vi "Corner Position to Bounds.vi"(10 "bottom right":T1, 11 "top left":T1) -> (3 "bounds":T2)   [LabVIEW 2010, in "NI_SE_Front Panel Layout.lvlib"]
uses:
  NI_SE_Front Panel Layout.lvlib
  <vilib>/Utility/miscctls.llb/LVRectTypeDef.ctl
  <vilib>/Utility/miscctls.llb/LVPointTypeDef.ctl
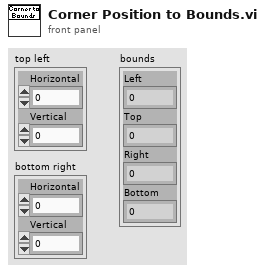
[diagram p1: front panel]
types:
  T1 = typedef "LVPointTypeDef.ctl" = cluster{"Horizontal":i16, "Vertical":i16}
  T2 = typedef "LVRectTypeDef.ctl" = cluster{"Left":i16, "Top":i16, "Right":i16, "Bottom":i16}
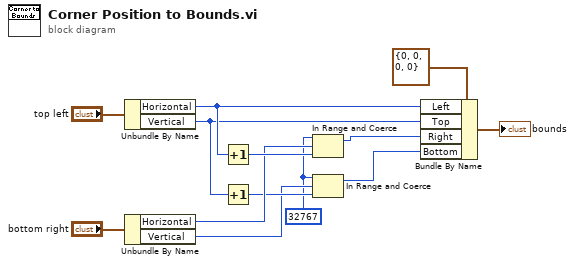
[diagram p0: block diagram]
diagram:
  w1 = i16 32767 ("upper limit")
  n1 = Unbundle By Name("top left") -> ("Horizontal"=w9:i16, "Vertical"=w5:i16)
  n2 = Unbundle By Name("bottom right") -> ("Horizontal"=w7:i16, "Vertical"=w3:i16)
  n3 = Increment(x=w9) -> (x+1=w8:i16)
  n4 = Increment(x=w5) -> (x+1=w4:i16)
  n5 = In Range and Coerce(upper limit=w1, x=w7, lower limit=w8) -> (coerced(x)=w6:i16)  [unwired: 1 out]
  n6 = In Range and Coerce(upper limit=w1, x=w3, lower limit=w4) -> (coerced(x)=w2:i16)  [unwired: 1 out]
  n7 = Bundle By Name(cluster=T2 {"Left"=0, "Top"=0, "Right"=0, "Bottom"=0} ("bounds"), "Left"=w9, "Top"=w5, "Right"=w6, "Bottom"=w2) -> (→"bounds":T2)
